vi "Read Last Waveform.vi"(8 "Error In":errorcluster, 10 "Channel":u8, 11 "reference in":refnum<class "PXIe-5172Ref.lvclass">) -> (0 "Error Out":errorcluster, 2 "Last Waveform":waveform(dbl), 3 "reference out":refnum<class "PXIe-5172Ref.lvclass">)   [LabVIEW 2023, in "PXIe-5172.lvlib" / "PXIe-5172Ref.lvclass"]
uses:
  PXIe-5172Ref.lvclass
  PXIe-5172.lvclass
  PXIe-5172Ref.lvclass/PXIe-5172Ref.ctl
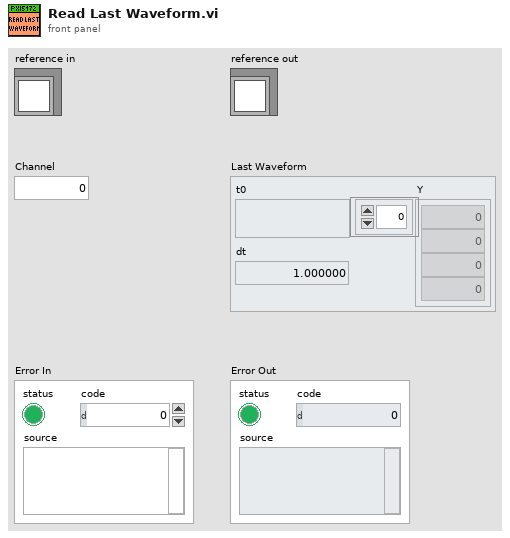
[diagram p1: front panel]
types:
  T1 = typedef "PXIe-5172.lvlib/PXIe-5172Ref.lvclass/ObjectAttributes.ctl" = cluster{"PXIe-5172.lvclass":refnum<class "PXIe-5172.lvclass">}
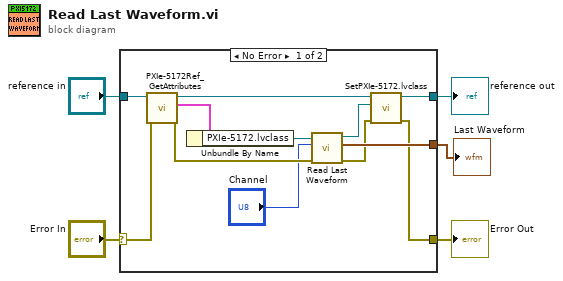
[diagram p0: block diagram]
diagram:
  n1 = case shown="No Error" "Error In" {
    selector: "Error In" -> [w17 w19]
    tunnel: [w6 w19] -> w4
    tunnel: [w9 w18] -> w2
    tunnel: "reference in" -> [w15 w18]
    tunnel: [w10 _] -> w1
    frame No Error {
      n2 = call "PXIe-5172Ref_GetAttributes.vi"("Error In"=w17, "reference in"=w15) -> ("Error Out"=w12:errorcluster, "Data"=w16:T1, "reference out"=w14:refnum<class "PXIe-5172Ref.lvclass">)  [unwired: 6 in, 1 out]
      n3 = Unbundle By Name(w16) -> ("PXIe-5172.lvclass"=w13:refnum<class "PXIe-5172.lvclass">)
      n4 = call-dynamic "Read Last Waveform.vi"("error in (no error)"=w12, "Channel"="Channel", "Scope Base in"=w13) -> ("error out"=w7:errorcluster, "Last Waveform"=w10:waveform(dbl), "Scope Base out"=w8:refnum<class "PXIe-5172.lvclass">)  [unwired: 6 in]
      n5 = call "SetPXIe-5172.lvclass.vi"("Error In"=w7, "PXIe-5172.lvclass"=w8, "reference in"=w14) -> ("Error Out"=w6:errorcluster, "reference out"=w9:refnum<class "PXIe-5172Ref.lvclass">)  [unwired: 7 in]
    }
    frame Error {
    }
  }
  "Error Out" <- w4
  "reference out" <- w2
  "Last Waveform" <- w1
